vi "files.vi"() -> ()   [LabVIEW 2015]
panel:
  in  "File Path Control":path
  in  "ActiveX Container":refnum<k7>(container)
  in  "PASSWORD":string
  in  "USER NAME":string
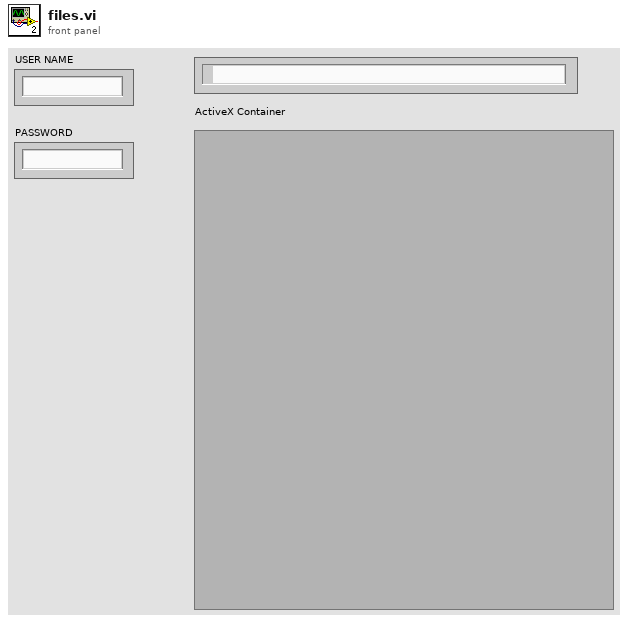
[diagram p1: front panel]
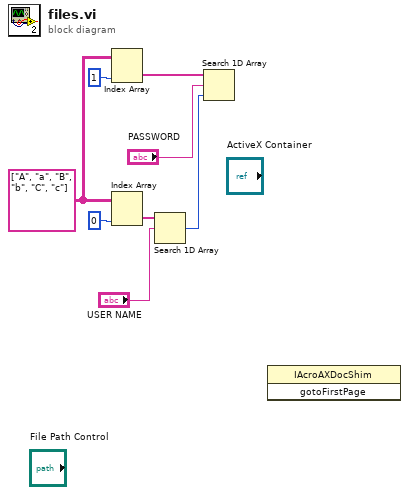
[diagram p0: block diagram]
diagram:
  w8 = string[][] [["A", "a"], ["B", "b"], ["C", "c"]]
  n1 = Index Array(array=w8, index (col)=1 ("disabled index (col)")) -> (element=w3:string[])  [unwired: 1 in]
  n2 = Index Array(array=w8, index (col)=0 ("disabled index (col)")) -> (element=w5:string[])  [unwired: 1 in]
  n3 = Search 1D Array(1D array=w5, element="USER NAME") -> (index of element=w2:i32)  [unwired: 1 in]
  n4 = Search 1D Array(1D array=w3, element="PASSWORD", start index (0)=w2) -> ()  [unwired: 1 out]
  n5 = invoke class="IAcroAXDocShim" method="gotoFirstPage"() -> ()  [unwired: 3 in, 3 out]
